vi "Error FLUSH.vi"(0 "Error Handler in":refnum<class "TLB` Error Handler.lvclass">, 5 "action queue in":refnum<queue>) -> (4 "Error Handler out":refnum<class "TLB` Error Handler.lvclass">, 15 "error out":errorcluster)   [LabVIEW 2023, in "TLB` InstStu GPlugin Template.lvlib" / "TLB` Error Handler.lvclass"]
doc: "<B>flush</B> existing action queue.\n\n<B>Input Parameters</B>\n\n<B>Error Handler in</B> identifies your session. <B>Error Handler in</B> is obtained from the Open.vi of this class.\n\n<B>action queue in</B> is a reference to a queue. Use the Create Action Queue function to obtain a queue reference. \n\n<B>Output Parameters</B>\n\n<B>Error Handler out</B> identifies your session. 'Error Handler out' is obtained from the Open.vi of this class.\n\n<B>error out</B> contains error information. This output provides standard error out functionality."
uses:
  TLB` Error Handler.lvclass
  Actions/System Action Element.ctl
  Actions/Actions.lvlib
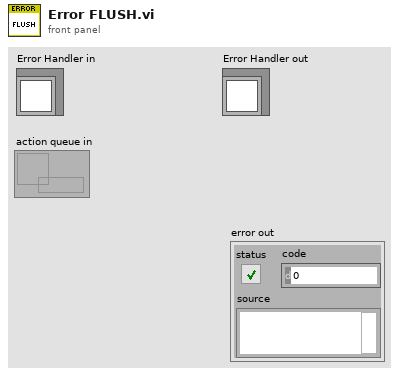
[diagram p1: front panel]
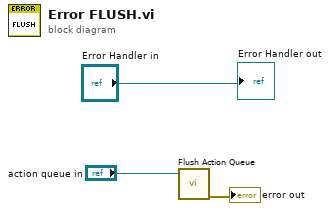
[diagram p0: block diagram]
diagram:
  n1 = call "Flush Action Queue.vi"("action queue in"="action queue in") -> ("error out"=→"error out":errorcluster)  [unwired: 12 in, 2 out]
  "Error Handler out" <- "Error Handler in"
